vi "Generate Pixel DVR.vi"(8 "Error In":errorcluster, 11 "Pixel In":refnum<class "Pixel.lvclass">) -> (0 "Error Out":errorcluster, 3 "Pixel Out":refnum<class "Pixel.lvclass">)   [LabVIEW 2019, in "Pixel.lvclass"]
uses:
  Pixel.lvclass
  Controls/Data.ctl
  Display Utilities/Public/Controls/2D Coordinates.ctl
  Pixel.lvclass/Pixel.ctl
  Display Utilities/Display Utilities.lvlib
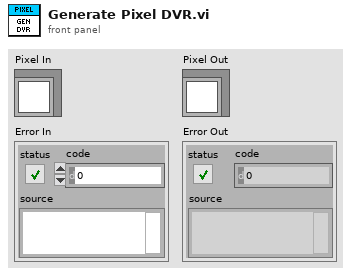
[diagram p1: front panel]
types:
  T1 = typedef "Pixel.lvclass/Data.ctl" = cluster{"Trace":i32, "Positions History":T2[]}
  T2 = typedef "Display Utilities.lvlib/2D Coordinates.ctl" = cluster{"X":i32, "Y":i32}
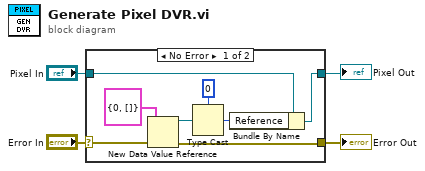
[diagram p0: block diagram]
diagram:
  n1 = case shown="No Error" "Error In" {
    selector: "Error In" -> [w12 w14]
    tunnel: "Pixel In" -> [w9 w13]
    tunnel: [w6 w14] -> w3
    tunnel: [w7 w13] -> w1
    frame No Error {
      n2 = New Data Value Reference(data value=T1 {"Trace"=0, "Positions History"=[]} ("Data"), error in=w12) -> (data value reference=w10:refnum<data-value>, error out=w6:errorcluster)
      n3 = Type Cast(type=u64 0, x=w10) -> (*(type *) &x=w8:u64)
      n4 = Bundle By Name(cluster=w9, "Reference"=w8) -> (w7:refnum<class "Pixel.lvclass">)
    }
    frame Error {
    }
  }
  "Error Out" <- w3
  "Pixel Out" <- w1
